vi "Waveform Data.vi"(8 "error in (no error)":errorcluster, 9 "Data Name Array":string[](array[string]), 10 "Data":waveform(dbl)[](array[waveform]), 11 "UI_Waveform in":refnum<class "UI_Waveform.lvclass">) -> (0 "error out":errorcluster, 3 "UI_Waveform out":refnum<class "UI_Waveform.lvclass">)   [LabVIEW 2021, in "UI_Waveform.lvclass"]
uses:
  UI_Waveform.lvclass
  UI_Waveform.lvclass/UI_Waveform.ctl
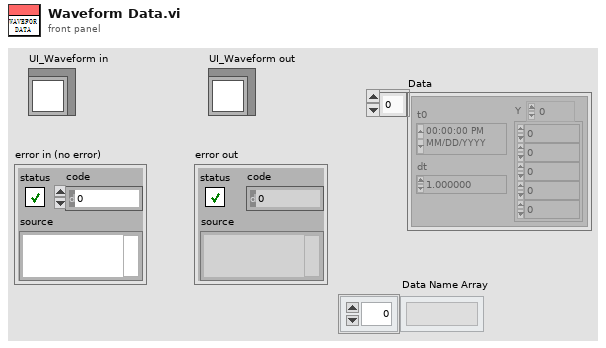
[diagram p1: front panel]
types:
  T1 = typedef "LVRectTypeDef.ctl" = cluster{"Left":i16, "Top":i16, "Right":i16, "Bottom":i16}
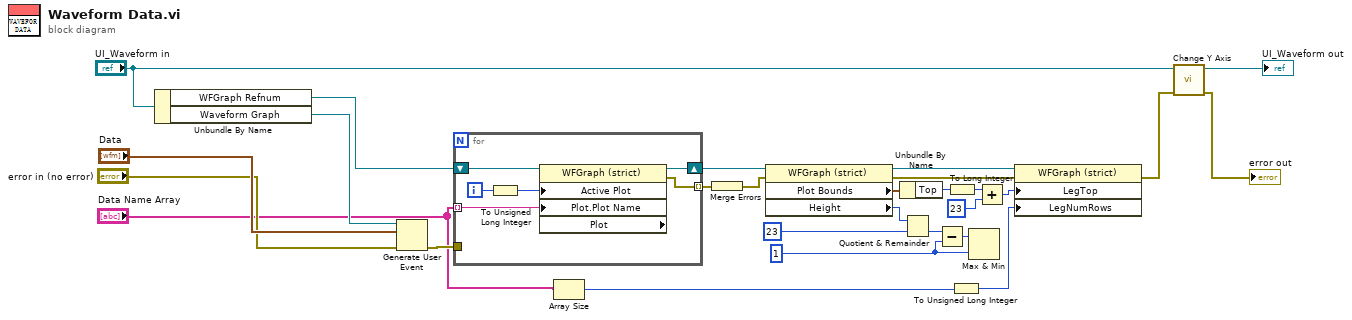
[diagram p0: block diagram]
diagram:
  w13 = u32 1 ("legend row holdoff")
  n1 = Unbundle By Name("UI_Waveform in") -> ("WFGraph Refnum"=w24:refnum<vi>, "Waveform Graph"=w27:refnum<user-event>)
  n2 = Generate User Event(user event=w27, event data cluster="Data", error in="error in (no error)") -> (error out=w23:errorcluster)  [unwired: 1 in, 1 out]
  n3 = for {
    tunnel: "Data Name Array" -> [w32] mode=indexing
    tunnel: w23 -> [_]
    shift-right: [w29] -> w10
    shift-left: w24 -> [w33]
    tunnel: [w28] -> w9 mode=indexing
    i -> [w31]
    n4 = To Unsigned Long Integer(number=w31) -> (unsigned 32bit integer=w30:u32)
    n5 = property class="WFGraph (strict)" props=["Active Plot", "Plot", "Plot Name", "Plot"](reference=w33, "Active Plot"=w30, "Plot.Plot Name"=w32) -> (reference out=w29:refnum<vi>, error out=w28:errorcluster)  [unwired: 1 in, 1 out]
  }
  n6 = Array Size(array="Data Name Array") -> (size(s)=w6:i32)
  n7 = Merge Errors(w9) -> (w8:errorcluster)
  n8 = property on="Property Node" class="WFGraph (strict)"(reference=w10, error in=w8) -> (reference out=w14:refnum<vi>, error out=w11:errorcluster, "Plot Bounds"=w18:T1, "Height"=w17:u32)
  n9 = Unbundle By Name(w18) -> ("Top"=w19:i16)
  n10 = Quotient & Remainder(x=w17, y=u32 23 ("legend row height")) -> (floor(x/y)=w15:u32)  [unwired: 1 out]
  n11 = Subtract(x=w15, y=w13) -> (x-y=w12:u32)
  n12 = To Long Integer(number=w19) -> (32bit integer=w22:i32)
  n13 = To Unsigned Long Integer(number=w6) -> (unsigned 32bit integer=w5:u32)
  n14 = Max & Min(x=w12, y=w13) -> ()  [unwired: 2 out]
  n15 = Add(x=w22, y=23) -> (x+y=w21:i32)
  n16 = property on="Property Node" class="WFGraph (strict)"(reference=w14, error in=w11, "LegTop"=w21, "LegNumRows"=w5) -> (error out=w2:errorcluster)  [unwired: 1 out]
  n17 = call "Change Y Axis.vi"("error in (no error)"=w2, "UI_Waveform in"="UI_Waveform in") -> ("error out"=→"error out":errorcluster, "UI_Waveform out"=→"UI_Waveform out":refnum<class "UI_Waveform.lvclass">)  [unwired: 8 in]
